vi "PH_AxisGUI_BaseClass.set i Attr.vi"(2 "error in (no error)":errorcluster, 3 "Instance Name":string) -> (0 "error out":errorcluster, 1 "i Attributes":T1)   [LabVIEW 2014, in "PH_AxisGUI_BaseClass.lvlib"]
uses:
  PH_AxisGUI_BaseClass.lvlib
  PH_AxisGUI_BaseClass.i attribute.ctl
  PH_AxisGUI_BaseClass.Axis Attributes.ctl
  PH_AxisGUI_BaseClass.Axis GUI Refs.ctl
  PH_Stepmotor_BaseClass/PH_Stepmotor_BaseClass.Axis Address.ctl
  PH_Stepmotor_BaseClass/PH_Stepmotor_BaseClass.Axis Settings.ctl
  PH_Stepmotor_BaseClass/PH_Stepmotor_BaseClass.Motor Type.ctl
  PH_Stepmotor_BaseClass/PH_Stepmotor_BaseClass.Axis Activity.ctl
  PH_Stepmotor_BaseClass/PH_Stepmotor_BaseClass.lvlib
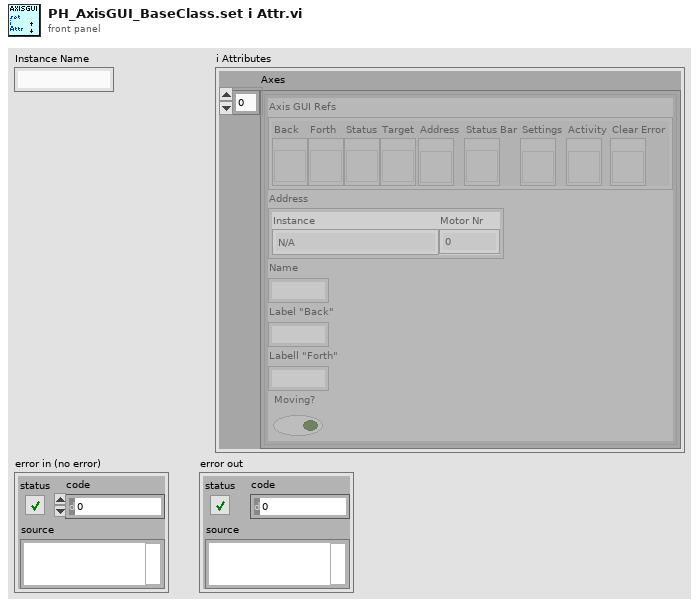
[diagram p1: front panel]
types:
  T1 = typedef "PH_AxisGUI_BaseClass.lvlib/PH_AxisGUI_BaseClass.i attribute.ctl" = cluster{"Axes":T2[]}
  T2 = typedef "PH_AxisGUI_BaseClass.lvlib/PH_AxisGUI_BaseClass.Axis Attributes.ctl" = cluster{"Axis GUI Refs":T3, "Address":T4, "Name":string, "Label \"Back\"":string, "Labell \"Forth\"":string, "Moving?":bool}
  T3 = typedef "PH_AxisGUI_BaseClass.lvlib/PH_AxisGUI_BaseClass.Axis GUI Refs.ctl" = cluster{"Back":refnum<vi>, "Forth":refnum<vi>, "Status":refnum<vi>, "Target":refnum<vi>, "Address":refnum<vi>, "Status Bar":refnum<vi>, "Settings":refnum<vi>, "Activity":refnum<vi>, "Clear Error":refnum<vi>}
  T4 = typedef "PH_Stepmotor_BaseClass.lvlib/PH_Stepmotor_BaseClass.Axis Address.ctl" = cluster{"Instance":string, "Motor Nr":i32}
  T5 = typedef "PH_AxisGUI_BaseClass.lvlib/PH_AxisGUI_BaseClass.Database Entry.ctl" = cluster{"Address":T4, "Name":string, "Label \"Back\"":string, "Labell \"Forth\"":string}
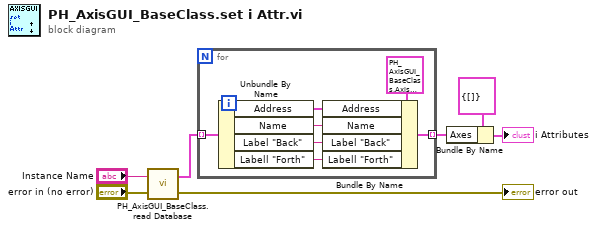
[diagram p0: block diagram]
diagram:
  n1 = call "PH_AxisGUI_BaseClass.read Database.vi"("error in (no error)"="error in (no error)", "DB Entry to read"="Instance Name") -> ("error out"=→"error out":errorcluster, "DB EntriesArray"=w2:T5[])
  n2 = for {
    tunnel: w2 -> [w14] mode=indexing
    tunnel: [w8] -> w1 mode=indexing
    n3 = Unbundle By Name(w14) -> ("Address"=w12:T4, "Name"=w11:string, "Label \"Back\""=w10:string, "Labell \"Forth\""=w9:string)
    n4 = Bundle By Name(cluster=T2 {"Axis GUI Refs"={"Back"=refnum, "Forth"=refnum, "Status"=refnum, "Target"=refnum, "Address"=refnum, "Status Bar"=refnum, "Settings"=refnum, "Activity"=refnum, "Clear Error"=refnum}, "Address"={"Instance"="N/A", "Motor Nr"=0}, "Name"="", "Label \"Back\""="", "Labell \"Forth\""="", "Moving?"=FALSE} ("Axis Attributes"), "Address"=w12, "Name"=w11, "Label \"Back\""=w10, "Labell \"Forth\""=w9) -> (w8:T2)
  }
  n5 = Bundle By Name(cluster=T1 {"Axes"=[]} ("CLASS.i attribute"), "Axes"=w1) -> (→"i Attributes":T1)
